vi "Set Switcher Relay Closed-Open2023.vi"(1 "Channel":i8 min=0 max=4 step=1, 2 "Group":i8 min=0 max=2, 3 "Slot":i8=1 min=1 max=5 step=1, 4 "Circuit":i8(ring) items=["CLOSED", "OPEN"], 5 "Device Configuration":T1={"Relay Type"=0, "GPIB Address"=6, "GPIB Card"=0} {"GPIB Card" min=0 max=30; "GPIB Address" min=0 max=30; "Relay Type" items=["HP3488A (44472A)", "HP34970A (34905A)"]}) -> (0 "Command Failed":bool)   [LabVIEW 2023]
doc: "This VI is used to open and close relays on a switcher.\n\nWhen connecting wires to this VI:\n\nTo close a relay, 'circuit' should be connected to '0'.\nTo open a relay, 'circuit' should be connected to '1'.\n\nCurrently supports:\n\nHP3488A (44472A)"
panel:
  # "Configuration"
  # "Settings"
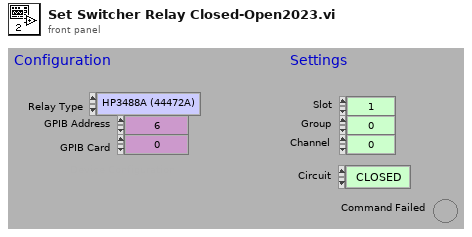
[diagram p1: front panel]
types:
  T1 = cluster{"Relay Type":i8, "GPIB Address":i8, "GPIB Card":i8}
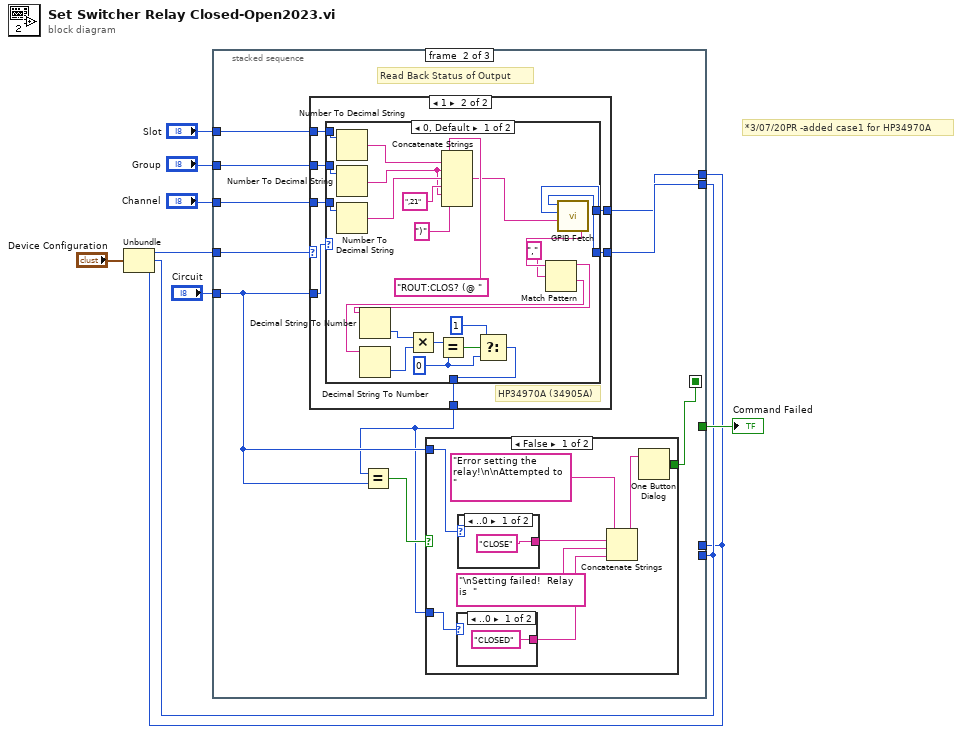
[diagram p0: block diagram]
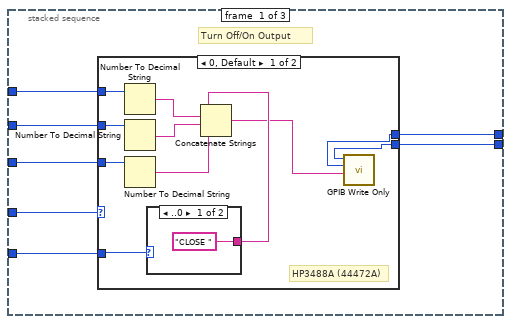
[diagram p2: hidden frame]
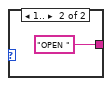
[diagram p3: hidden frame]
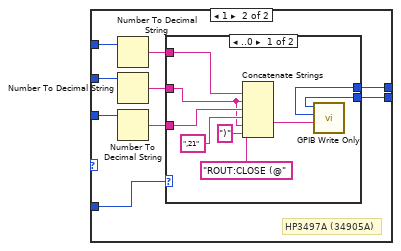
[diagram p4: hidden frame]
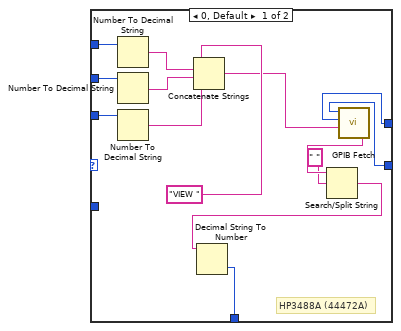
[diagram p6: hidden frame]
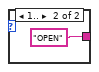
[diagram p8: hidden frame]
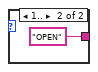
[diagram p9: hidden frame]
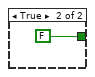
[diagram p10: hidden frame]
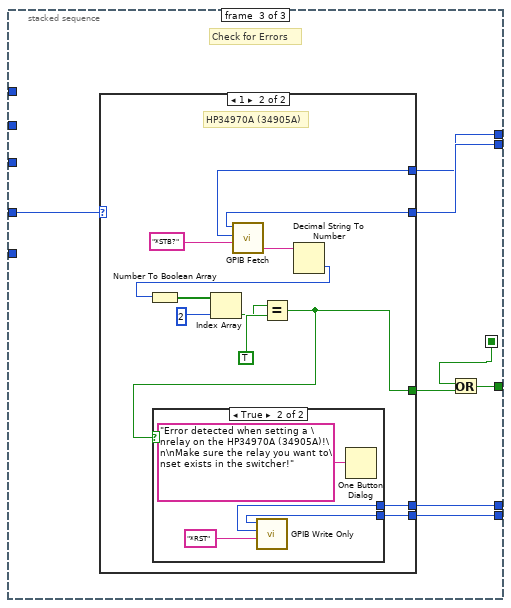
[diagram p11: hidden frame]
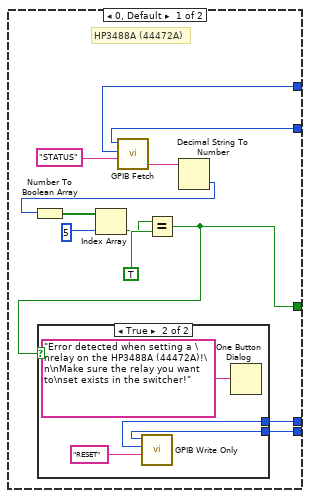
[diagram p12: hidden frame]
diagram:
  # "*3/07/20PR -added case1 for HP34970A"
  n1 = Unbundle("Device Configuration") -> ("Relay Type"=w6:i8, "GPIB Address"=w2:i8, "GPIB Card"=w1:i8)
  n2 = stacked-sequence {
    seq-local: [_ w49 _] -> [_ _ w120]
    tunnel: "Slot" -> [w14 w55 _]
    tunnel: w6 -> [w15 w52 w121]
    tunnel: "Circuit" -> [w16 w50 _]
    tunnel: w2 -> [w12 w57 w123]
    tunnel: w1 -> [w13 w51 w122]
    tunnel: "Channel" -> [w11 w53 _]
    tunnel: "Group" -> [w10 w54 _]
    tunnel: [_ _ w118] -> w3
    tunnel: w2 -> [_ _ w117]
    tunnel: w1 -> [_ _ w116]
    frame #0 {
      # "Turn Off/On Output"
      n3 = case shown="0, Default" w15 {
        tunnel: w14 -> [w27 w38]
        tunnel: w16 -> [w21 w35]
        tunnel: w13 -> [w20 w34]
        tunnel: w12 -> [w19 w33]
        tunnel: w11 -> [w26 w37]
        tunnel: w10 -> [w25 w36]
        frame 0, Default {
          # "HP3488A (44472A)"
          n4 = Number To Decimal String(number=w27) -> (decimal integer string=w24:string)  [unwired: 1 in]
          n5 = Number To Decimal String(number=w25) -> (decimal integer string=w23:string)  [unwired: 1 in]
          n6 = Number To Decimal String(number=w26) -> (decimal integer string=w22:string)  [unwired: 1 in]
          n7 = case shown="..0" w21 {
            tunnel: ["CLOSE " "OPEN "] -> w18
            frame ..0 {
            }
            frame 1.. {
            }
          }
          n8 = Concatenate Strings(w18, w24, w23, w22) -> (w17:string)
          n9 = call "GPIB Write Only.vi"("Command String"=w17, "GPIB Card"=w20, "GPIB Address"=w19) -> ()  [unwired: 3 in, 1 out]
        }
        frame 1 {
          # "HP3497A (34905A)"
          n10 = Number To Decimal String(number=w38) -> (decimal integer string=w32:string)  [unwired: 1 in]
          n11 = Number To Decimal String(number=w36) -> (decimal integer string=w31:string)  [unwired: 1 in]
          n12 = Number To Decimal String(number=w37) -> (decimal integer string=w30:string)  [unwired: 1 in]
          n13 = case shown="..0" w35 {
            tunnel: w34 -> [w47 _]
            tunnel: w33 -> [w46 _]
            tunnel: w32 -> [w43 _]
            tunnel: w31 -> [w40 _]
            tunnel: w30 -> [w42 _]
            frame ..0 {
              n14 = Concatenate Strings("ROUT:CLOSE (@", w43, w40, w42, ",21" ("string"), w40, ")" ("string")) -> (w45:string)
              n15 = call "GPIB Write Only.vi"("Command String"=w45, "GPIB Card"=w47, "GPIB Address"=w46) -> ()  [unwired: 3 in, 1 out]
            }
            frame 1.. {
            }
          }
        }
      }
    }
    frame #1 {
      # "Read Back Status of Output"
      n16 = case shown="1" w52 {
        tunnel: w55 -> [w71 w78]
        tunnel: w50 -> [_ w72]
        tunnel: w53 -> [w70 w76]
        tunnel: w54 -> [w69 w77]
        tunnel: w51 -> [w64 w74]
        tunnel: w57 -> [w63 w75]
        tunnel: [w58 w73] -> w48
        frame 0, Default {
          # "HP3488A (44472A)"
          n17 = Number To Decimal String(number=w71) -> (decimal integer string=w68:string)  [unwired: 1 in]
          n18 = Number To Decimal String(number=w69) -> (decimal integer string=w67:string)  [unwired: 1 in]
          n19 = Number To Decimal String(number=w70) -> (decimal integer string=w66:string)  [unwired: 1 in]
          n20 = Concatenate Strings("VIEW ", w68, w67, w66) -> (w62:string)
          n21 = call "GPIB Fetch.vi"("Command String"=w62, "GPIB Card"=w64, "GPIB Address"=w63) -> ("Characters Read"=w61:string)  [unwired: 1 in, 2 out]
          n22 = Search/Split String(string=w61, search string/char (-)=" ") -> (match + rest of string=w59:string)  [unwired: 1 in, 2 out]
          n23 = Decimal String To Number(string=w59) -> (number=w58:i32)  [unwired: 2 in, 1 out]
        }
        frame 1 {
          # "HP34970A (34905A)"
          n24 = case shown="0, Default" w72 {
            selector: w72 -> [_ w102]
            tunnel: w78 -> [w84 _]
            tunnel: w77 -> [w83 _]
            tunnel: w76 -> [w82 _]
            tunnel: w75 -> [w81 _]
            tunnel: w74 -> [w80 _]
            tunnel: [w79 w102] -> w73
            frame 0, Default {
              w85 = 0 ("y")
              n25 = Number To Decimal String(number=w84) -> (decimal integer string=w101:string)  [unwired: 1 in]
              n26 = Number To Decimal String(number=w83) -> (decimal integer string=w94:string)  [unwired: 1 in]
              n27 = Number To Decimal String(number=w82) -> (decimal integer string=w100:string)  [unwired: 1 in]
              n28 = Concatenate Strings("ROUT:CLOS? (@ ", w101, w94, w100, ",21" ("string"), w94, ")" ("string")) -> (w98:string)
              n29 = call "GPIB Fetch.vi"("Command String"=w98, "GPIB Card"=w80, "GPIB Address"=w81) -> ("Characters Read"=w97:string)  [unwired: 1 in, 2 out]
              n30 = Match Pattern(string=w97, regular expression=",") -> (before substring=w91:string, after substring=w92:string)  [unwired: 1 in, 2 out]
              n31 = Decimal String To Number(string=w91) -> (number=w90:i32)  [unwired: 2 in, 1 out]
              n32 = Decimal String To Number(string=w92) -> (number=w89:i32)  [unwired: 2 in, 1 out]
              n33 = Multiply(x=w90, y=w89) -> (x*y=w88:i32)
              n34 = Equal?(x=w88, y=w85) -> (x = y?=w87:bool)
              n35 = Select(t=i8 1, s=w87, f=w85) -> (s? t:f=w79:i32)
            }
            frame 1 {
            }
          }
        }
      }
      n36 = Equal?(x=w48, y=w50) -> (x = y?=w56:bool)
      n37 = case shown="False" w56 {
        tunnel: [w109 FALSE] -> w49
        tunnel: w48 -> [w108 _]
        tunnel: w50 -> [w107 _]
        frame False {
          n38 = case shown="..0" w108 {
            tunnel: ["CLOSED" "OPEN"] -> w103
            frame ..0 {
            }
            frame 1.. {
            }
          }
          n39 = case shown="..0" w107 {
            tunnel: ["CLOSE" "OPEN"] -> w105
            frame ..0 {
            }
            frame 1.. {
            }
          }
          n40 = Concatenate Strings("Error setting the relay!\n\nAttempted to  ", w105, "\nSetting failed!  Relay is  ", w103) -> (w110:string)
          n41 = One Button Dialog(message=w110) -> (true=w109:bool)  [unwired: 1 in]
        }
        frame True {
        }
      }
    }
    frame #2 {
      # "Check for Errors"
      n42 = case shown="1" w121 {
        tunnel: w122 -> [w134 w150]
        tunnel: w123 -> [w133 w149]
        tunnel: [w126 w142] -> w119
        tunnel: w117 -> [w125 w141]
        tunnel: w116 -> [w124 w140]
        frame 0, Default {
          # "HP3488A (44472A)"
          n43 = call "GPIB Fetch.vi"("Command String"="STATUS", "GPIB Card"=w134, "GPIB Address"=w133) -> ("Characters Read"=w132:string)  [unwired: 1 in, 2 out]
          n44 = Decimal String To Number(string=w132) -> (number=w131:i32)  [unwired: 2 in, 1 out]
          n45 = Number To Boolean Array(number=w131) -> (Boolean array=w130:bool[])
          n46 = Index Array(array=w130, index=5) -> (element=w127:bool)
          n47 = Equal?(x=w127, y=TRUE) -> (x = y?=w126:bool)
          n48 = case shown="True" w126 {
            tunnel: w125 -> [_ w138]
            tunnel: w124 -> [_ w137]
            frame False {
            }
            frame True {
              n49 = call "GPIB Write Only.vi"("Command String"="RESET", "GPIB Card"=w137, "GPIB Address"=w138) -> ()  [unwired: 3 in, 1 out]
              n50 = One Button Dialog(message="Error detected when setting a \nrelay on the HP3488A (44472A)!\n\nMake sure the relay you want to\nset exists in the switcher!") -> ()  [unwired: 1 in, 1 out]
            }
          }
        }
        frame 1 {
          # "HP34970A (34905A)"
          n51 = call "GPIB Fetch.vi"("Command String"="*STB?", "GPIB Card"=w150, "GPIB Address"=w149) -> ("Characters Read"=w148:string)  [unwired: 1 in, 2 out]
          n52 = Decimal String To Number(string=w148) -> (number=w147:i32)  [unwired: 2 in, 1 out]
          n53 = Number To Boolean Array(number=w147) -> (Boolean array=w146:bool[])
          n54 = Index Array(array=w146, index=2) -> (element=w143:bool)
          n55 = Equal?(x=w143, y=TRUE) -> (x = y?=w142:bool)
          n56 = case shown="True" w142 {
            tunnel: w141 -> [_ w154]
            tunnel: w140 -> [_ w153]
            frame False {
            }
            frame True {
              n57 = call "GPIB Write Only.vi"("Command String"="*RST", "GPIB Card"=w153, "GPIB Address"=w154) -> ()  [unwired: 3 in, 1 out]
              n58 = One Button Dialog(message="Error detected when setting a \nrelay on the HP34970A (34905A)!\n\nMake sure the relay you want to\nset exists in the switcher!") -> ()  [unwired: 1 in, 1 out]
            }
          }
        }
      }
      n59 = Or(x=w120, y=w119) -> (x .or. y?=w118:bool)
    }
  }
  "Command Failed" <- w3
